vi "testRemoveLastElement.vi"(8 "error in (no error)":errorcluster, 11 "TestCase in":refnum<class "ListImp_Empty.lvclass">) -> (0 "error out":errorcluster, 3 "TestCase out":refnum<class "ListImp_Empty.lvclass">)   [LabVIEW 2013, in "ListImp_Empty.lvclass"]
uses:
  ListImp_Empty.lvclass
  ListImp_Empty.lvclass/ListImp_Empty.ctl
  source/LapDog.Collections.Lists/ListImp/ListImp.lvclass
  <vilib>/addons/_JKI Toolkits/VI Tester/TestCase.llb/TestCase.lvclass
  UnitTestComparisons/UnitTestComparisons.lvlib
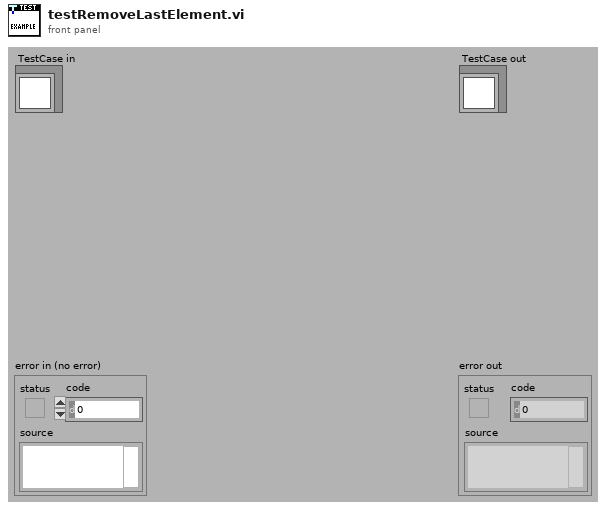
[diagram p1: front panel]
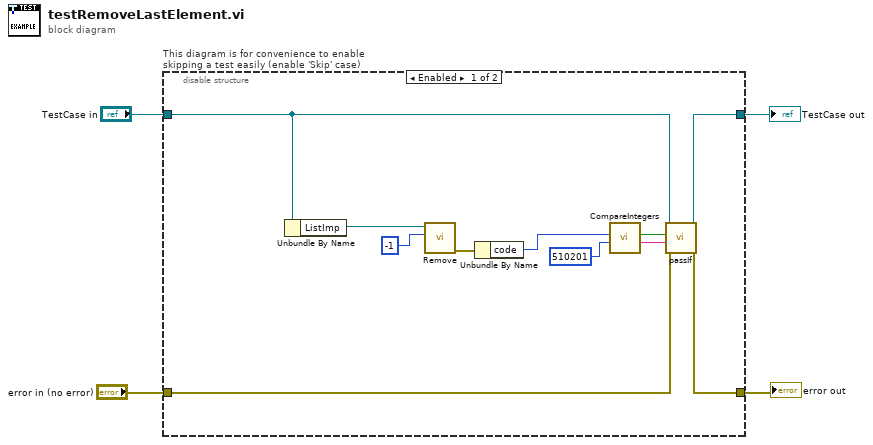
[diagram p0: block diagram]
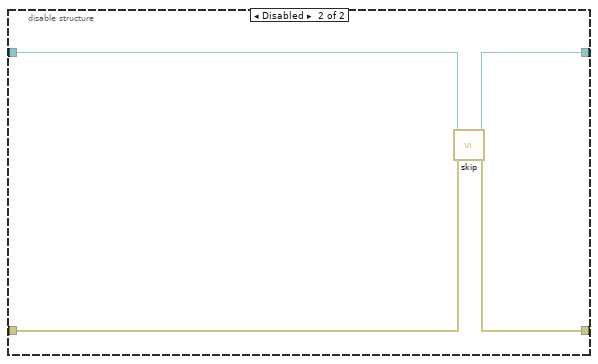
[diagram p2: hidden frame]
diagram:
  n1 = disable-structure "This diagram is for convenience to enable skipping a test easily (enable 'Skip' case)" shown="Enabled" {
    disable-tunnel: "TestCase in" -> [w12 w19]
    disable-tunnel: [w15 w17] -> w1
    disable-tunnel: [w14 w18] -> w3
    disable-tunnel: "error in (no error)" -> [w13 w16]
    frame Enabled {
      n2 = Unbundle By Name(w12) -> ("ListImp"=w6:refnum<class "ListImp.lvclass">)
      n3 = call-dynamic "Remove.vi"("Index"=-1, "ListImp in"=w6) -> ("error out"=w8:errorcluster)  [unwired: 7 in, 2 out]
      n4 = Unbundle By Name(w8) -> ("code"=w7:i32)
      n5 = call "CompareIntegers.vi"("Expected Value"=510201, "Actual Value"=w7) -> ("Message"=w10:string, "Equal?"=w11:bool)  [unwired: 8 in]
      n6 = call-dynamic "passIf.vi"("error in (no error)"=w13, "message (\"\")"=w10, "pass"=w11, "TestCase in"=w12) -> ("error out"=w14:errorcluster, "TestCase out"=w15:refnum<class "ListImp_Empty.lvclass">)  [unwired: 6 in]
    }
    frame Disabled {
      # "skip test result while test is under development"
      n7 = call <vilib>:"skip.vi"("error in (no error)"=w16, "TestCase in"=w19) -> ("error out"=w18:errorcluster, "TestCase out"=w17:refnum<class "ListImp_Empty.lvclass">)  [unwired: 8 in]
    }
  }
  "error out" <- w3
  "TestCase out" <- w1
